vi "Extract Tagged LLP Packets from Raw Data.vi"(0 "tagged packet data block":u8[](array[numeric]), 5 "block start packet index":i64, 7 "packet range upper":i64, 9 "packet range lower":i64) -> (4 "tagged packets":T1[](array[typedef]), 6 "block end packet index":i64, 8 "block bytes parsed":u32)   [LabVIEW 2023, in "GettingStarted_Common_148X_Host.lvlib"]
uses:
  GettingStarted_Common_148X_Host.lvlib
  <instrlib>/FlexRIO/CSI-2/v2/Host/Types/Host Tagged LLP Packet.ctl
  <instrlib>/FlexRIO/CSI-2/v2/Host/Types/Host LLP Packet Tag.ctl
  <instrlib>/FlexRIO/CSI-2/v2/Host/Types/Host LLP Packet Timestamp.ctl
  <instrlib>/FlexRIO/CSI-2/v2/FPGA/Types/Timestamp ID.ctl
  <instrlib>/FlexRIO/CSI-2/v2/Host/Types/Host LLP Packet Size.ctl
  <instrlib>/FlexRIO/CSI-2/v2/Host/Types/Host LLP Packet.ctl
  <instrlib>/FlexRIO/CSI-2/v2/FPGA/Types/LLP Packet Header.ctl
  <instrlib>/FlexRIO/CSI-2/v2/FPGA/Types/LLP Packet Footer.ctl
  <instrlib>/FlexRIO/CSI-2/v2/FPGA/Types/Raw Timestamp.ctl
  <instrlib>/FlexRIO/CSI-2/v2/Host/subVIs/Convert Raw Timestamp to LLP Packet Timestamp.vi
  <instrlib>/FlexRIO/CSI-2/v2/Host/NI CSI-2 API Host v2.lvlib
  <instrlib>/FlexRIO/CSI-2/v2/FPGA/NI CSI-2 API FPGA v2.lvlib
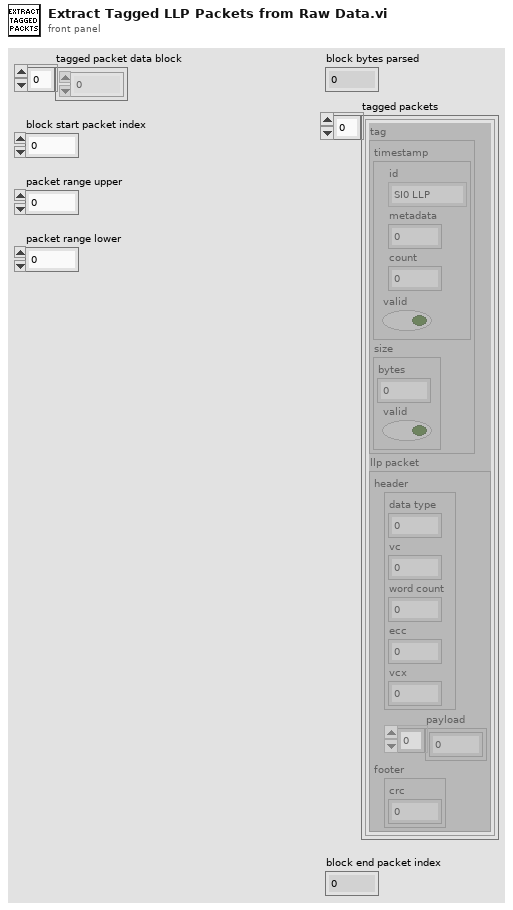
[diagram p1: front panel]
types:
  T1 = typedef "NI CSI-2 API Host v2.lvlib/Host Tagged LLP Packet.ctl" = cluster{"tag":T2, "llp packet":T6}
  T2 = typedef "NI CSI-2 API Host v2.lvlib/Host LLP Packet Tag.ctl" = cluster{"timestamp":T3, "size":T5}
  T3 = typedef "NI CSI-2 API Host v2.lvlib/Host LLP Packet Timestamp.ctl" = cluster{"valid":bool, "count":u64, "id":T4, "metadata":u8}
  T4 = typedef "NI CSI-2 API FPGA v2.lvlib/Timestamp ID.ctl" = enum8{"SI0 LLP", "SI1 LLP", "SI2 LLP", "SI3 LLP", "SI4 LLP", "SI5 LLP", "SI6 LLP", "SI7 LLP", "SO0 LLP", "SO1 LLP", "SO2 LLP", "SO3 LLP", "SO4 LLP", "SO5 LLP", "SO6 LLP", "SO7 LLP", "Ser0 GPIO Bank", "Ser1 GPIO Bank", "Ser2 GPIO Bank", "Ser3 GPIO Bank", "Ser4 GPIO Bank", "Ser5 GPIO Bank", "Ser6 GPIO Bank", "Ser7 GPIO Bank", "Des0 GPIO Bank", "Des1 GPIO Bank", "Des2 GPIO Bank", "Des3 GPIO Bank", "Des4 GPIO Bank", "Des5 GPIO Bank", "Des6 GPIO Bank", "Des7 GPIO Bank", "User0", "User1", "User2", "User3", "User4", "User5", "User6", "User7", "User8", "User9", "User10", "User11", "User12", "User13", "User14", "User15", "User16", "User17", "User18", "User19", "User20", "User21", "User22", "User23", "User24", "User25", "User26", "User27", "User28", "User29", "User30", "User31"}
  T5 = typedef "NI CSI-2 API Host v2.lvlib/Host LLP Packet Size.ctl" = cluster{"bytes":u32, "valid":bool}
  T6 = typedef "NI CSI-2 API Host v2.lvlib/Host LLP Packet.ctl" = cluster{"header":T7, "payload":u8[], "footer":T8}
  T7 = typedef "NI CSI-2 API FPGA v2.lvlib/LLP Packet Header.ctl" = cluster{"word count":u16, "ecc":fxp<+,6,6>, "vcx":fxp<+,2,2>, "data type":fxp<+,6,6>, "vc":fxp<+,2,2>}
  T8 = typedef "NI CSI-2 API FPGA v2.lvlib/LLP Packet Footer.ctl" = cluster{"crc":u16}
  T9 = typedef "NI CSI-2 API FPGA v2.lvlib/Raw Timestamp.ctl" = cluster{"timestamp":u64, "valid":bool}
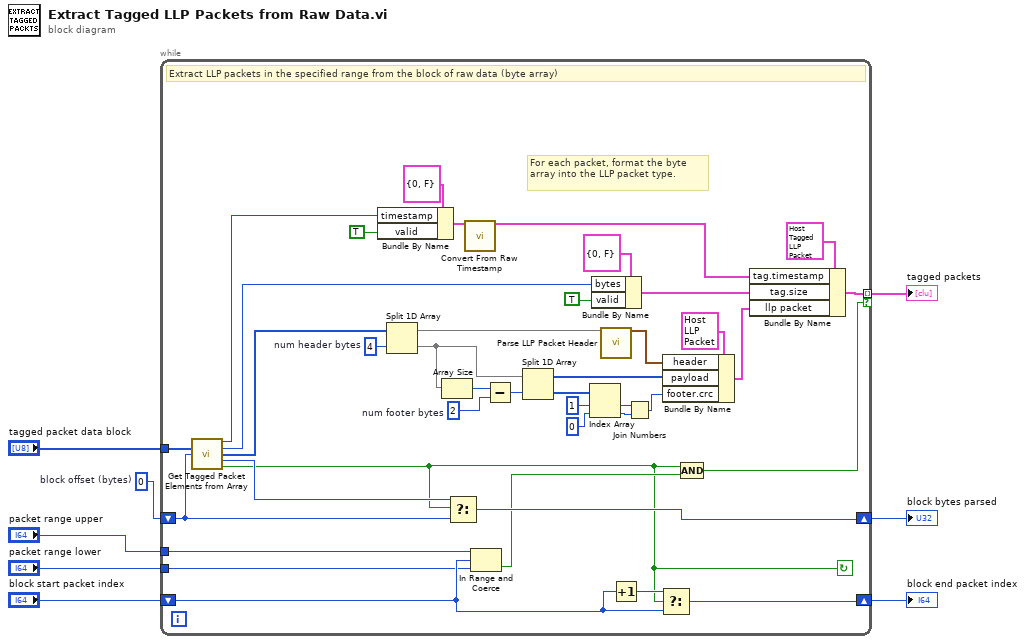
[diagram p0: block diagram]
diagram:
  w1 = u32 0  # block offset (bytes)
  n1 = while {
    tunnel: "tagged packet data block" -> [w12]
    shift-right: [w29] -> w8
    shift-left: w1 -> [w11]
    tunnel: [w30] -> w2 mode=indexing if=w15
    shift-right: [w26] -> w7
    shift-left: "block start packet index" -> [w24]
    tunnel: "packet range lower" -> [w23]
    tunnel: "packet range upper" -> [w9]
    stop <- w10 continue-if-true
    w46 = 2  # num footer bytes
    w48 = 4  # num header bytes
    # "For each packet, format the byte array into the LLP packet type."
    # "Extract LLP packets in the specified range from the block of raw data (byte array)"
    n2 = call "Get Tagged Packet Elements from Array.vi"("tagged packet data in"=w12, "tagged packet offset"=w11) -> ("packet timestamp"=w36:u64, "packet data length (bytes)"=w17:u32, "packet data"=w14:u8[], "total tagged packet size (bytes)"=w13:u32, "valid packet data?"=w10:bool)  [unwired: 9 in]
    n3 = Bundle By Name(cluster=T9 {"timestamp"=0, "valid"=FALSE} ("raw timestamp"), "timestamp"=w36, "valid"=TRUE) -> (w34:T9)
    n4 = Split 1D Array(array=w14, index=w48) -> (first subarray=w37:u8[], second subarray=w45:u8[])
    n5 = Array Size(array=w45) -> (size(s)=w47:i32)
    n6 = Select(t=w13, s=w10, f=w11) -> (s? t:f=w29:u32)
    n7 = call-poly <instrlib>:"Convert From Raw Timestamp.vi"("raw timestamp"=w34) -> ("llp packet timestamp"=w31:T3)  [unwired: 14 in]
    n8 = In Range and Coerce(upper limit=w9, x=w24, lower limit=w23) -> (In Range?=w16:bool)  [unwired: 1 out]
    n9 = Subtract(x=w47, y=w46) -> (x-y=w44:i32)
    n10 = Split 1D Array(array=w45, index=w44) -> (first subarray=w22:u8[], second subarray=w38:u8[])
    n11 = Index Array(array=w38, index #1=1 ("index"), index #2=0 ("index")) -> (element #1=w28:u8, element #2=w27:u8)
    n12 = Bundle By Name(cluster=T5 {"bytes"=0, "valid"=FALSE} ("host llp packet size"), "bytes"=w17, "valid"=TRUE) -> (w20:T5)
    n13 = call <instrlib>:"Parse LLP Packet Header.vi"("data"=w37) -> ("header"=w42:T7)  [unwired: 13 in, 1 out]
    n14 = Increment(x=w24) -> (x+1=w25:i64)
    n15 = Join Numbers(hi=w28, lo=w27) -> ((hi.lo)=w39:u16)
    n16 = Select(t=w25, s=w10, f=w24) -> (s? t:f=w26:i64)
    n17 = Bundle By Name(cluster=T6 {"header"={"word count"=0, "ecc"=0.0, "vcx"=0.0, "data type"=0.0, "vc"=0.0}, "payload"=[], "footer"={"crc"=0}}, "header"=w42, "payload"=w22, "footer.crc"=w39) -> (w21:T6)
    n18 = Compound Arithmetic op=AND(w10, w16) -> (w15:bool)
    n19 = Bundle By Name(cluster=T1 {"tag"={"timestamp"={"valid"=FALSE, "count"=0, "id"=enum."SI0 LLP", "metadata"=0}, "size"={"bytes"=0, "valid"=FALSE}}, "llp packet"={"header"={"word count"=0, "ecc"=0.0, "vcx"=0.0, "data type"=0.0, "vc"=0.0}, "payload"=[], "footer"={"crc"=0}}} ("host tagged llp packet"), "tag.timestamp"=w31, "tag.size"=w20, "llp packet"=w21) -> (w30:T1)
  }
  "block bytes parsed" <- w8
  "block end packet index" <- w7
  "tagged packets" <- w2
